vi "SingleButtonDetect.vi"(8 "Reset":bool, 11 "Buttons":bool[](array[boolean])) -> (3 "Pressed Index":i32)   [LabVIEW 2017]
uses:
  <userlib>/836-Library/Logic/Logic_Support/SingleButtonDetectStates.ctl
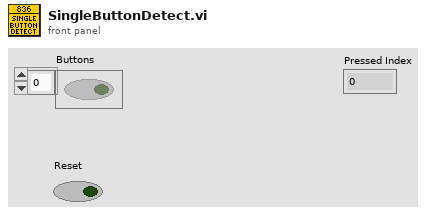
[diagram p1: front panel]
types:
  T1 = typedef "SingleButtonDetectStates.ctl" = enum16{"Idle", "Reset", "Press Detected"}
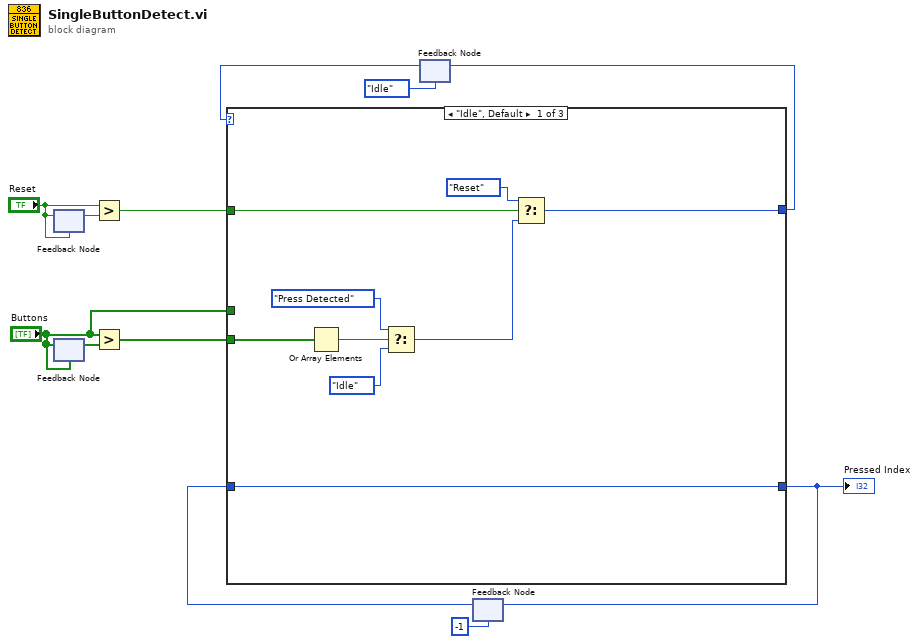
[diagram p0: block diagram]
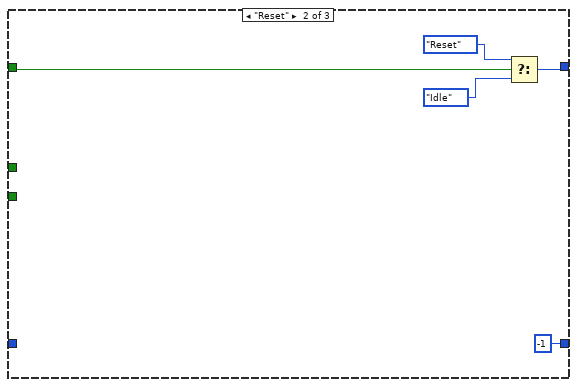
[diagram p2: hidden frame]
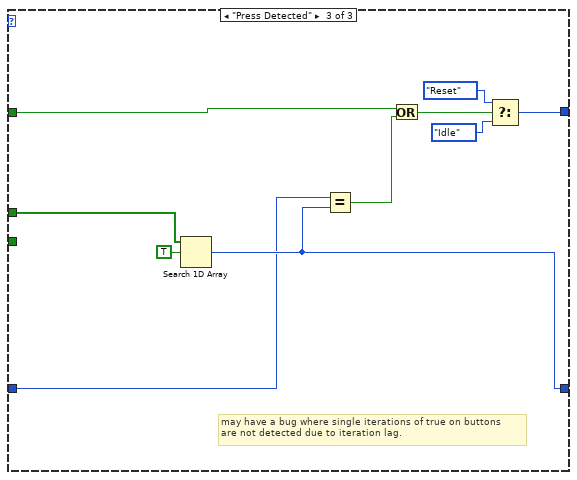
[diagram p3: hidden frame]
diagram:
  n1 = feedback-in #1("Reset") -> ()
  n2 = feedback #1("Reset") -> (w11:bool)
  n3 = feedback-in #2("Buttons") -> ()
  n4 = feedback #2("Buttons") -> (w9:bool[])
  n5 = Greater?(x="Reset", y=w11) -> (0:w6:bool)
  n6 = Greater?(x="Buttons", y=w9) -> (0:w7:bool[])
  n7 = feedback #3(SingleButtonDetectStates."Idle") -> (w8:T1)
  n8 = feedback #4(-1) -> (w4:i32)
  n9 = case shown="\"Idle\", Default" w8 {
    tunnel: w7 -> [w21 _ _]
    tunnel: w6 -> [w17 w25 w34]
    tunnel: [w14 w22 w35] -> w2
    tunnel: [w13 -1 w29] -> w3
    tunnel: w4 -> [w13 _ w28]
    tunnel: "Buttons" -> [_ _ w31]
    frame "Idle", Default {
      n10 = Or Array Elements(Boolean array=w21) -> (logical OR=w20:bool)
      n11 = Select(t=SingleButtonDetectStates."Press Detected", s=w20, f=SingleButtonDetectStates."Idle") -> (s? t:f=w16:T1)
      n12 = Select(t=SingleButtonDetectStates."Reset", s=w17, f=w16) -> (s? t:f=w14:T1)
    }
    frame "Reset" {
      n13 = Select(t=SingleButtonDetectStates."Reset", s=w25, f=SingleButtonDetectStates."Idle") -> (s? t:f=w22:T1)
    }
    frame "Press Detected" {
      # "may have a bug where single iterations of true on buttons\nare not detected due to iteration lag."
      n14 = Search 1D Array(1D array=w31, element=TRUE) -> (index of element=w29:i32)  [unwired: 1 in]
      n15 = Equal?(x=w28, y=w29) -> (x = y?=w27:bool)
      n16 = Or(x=w34, y=w27) -> (x .or. y?=w30:bool)
      n17 = Select(t=SingleButtonDetectStates."Reset", s=w30, f=SingleButtonDetectStates."Idle") -> (s? t:f=w35:T1)
    }
  }
  "Pressed Index" <- w3
  n18 = feedback-in #3(w2) -> ()
  n19 = feedback-in #4(w3) -> ()
